vi "setRowsColor.vi"(8 "error in (no error)":errorcluster, 10 "rowsColor":u32[](array[numeric]), 11 "reference in":refnum<class "excelFile.lvclass">) -> (0 "error out":errorcluster, 3 "reference out":refnum<class "excelFile.lvclass">)   [LabVIEW 2016, in "excelFile.lvclass"]
uses:
  excelFile.lvclass
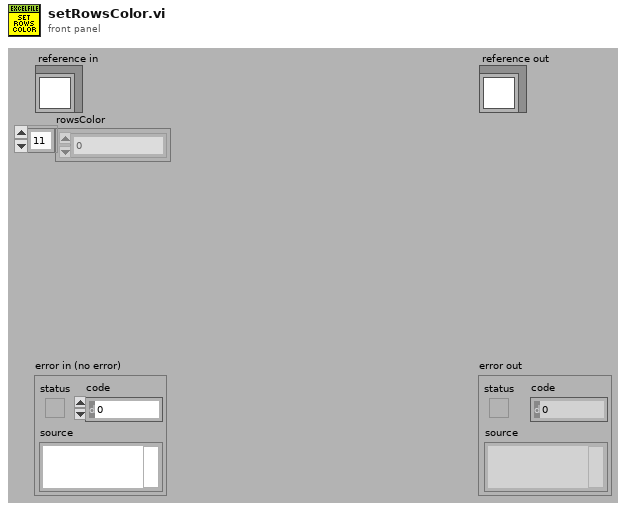
[diagram p1: front panel]
types:
  T1 = typedef "excelFile.lvclass/ObjectAttributesRef.ctl" = refnum<data-value>
  T2 = typedef "excelFile.lvclass/ObjectAttributes.ctl" = cluster{"MyAttribute":dbl, "path":string, "Refnum Excel":cluster{"Excel._Application":refnum<k7>, "Workbooks":refnum<k7>, "Open":refnum<k7>}, "data":string[][][], "save":bool, "fileType":T3, "rowsColor":u32[], "python_ref":refnum<class "python.lvclass">, "items_rows":i32[], "excel_range":i32[][], "TSR":cluster{"number":string, "TSR_path":path, "service_path":path, "email_to":string}, "excel_already_opened?":bool, "file_already_opened?":bool, "excel_protected_opened?":bool, "Refnum Cluster Worksheets":cluster{"Excel._Application":refnum<k7>, "Workbooks":refnum<k7>, "Open":refnum<k7>, "Worksheets":refnum<k7>, "Excel._Worksheet":refnum<k7>}, "#_rows_defective":i32, "#_rows_spare":i32}
  T3 = typedef "excelFile.lvclass/fileType.ctl" = enum16{"devices", "items", "partsTracking", "TSR"}
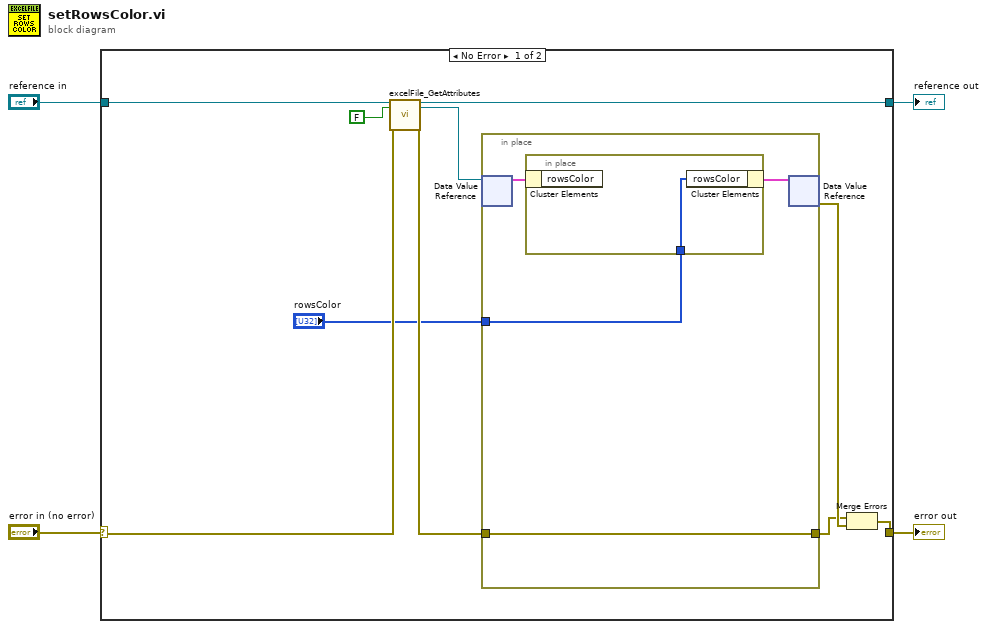
[diagram p0: block diagram]
diagram:
  n1 = case shown="No Error" "error in (no error)" {
    selector: "error in (no error)" -> [w9 w21]
    tunnel: [w14 w21] -> w3
    tunnel: [w7 w20] -> w1
    tunnel: "reference in" -> [w11 w20]
    frame No Error {
      n2 = call "excelFile_GetAttributes.vi"("reference in"=w11, "return data? (T)"=FALSE, "error in (no error)"=w9) -> ("reference out"=w7:refnum<class "excelFile.lvclass">, "attributes ref"=w6:T1, "error out"=w8:errorcluster)  [unwired: 13 in, 1 out]
      n3 = in-place {
        in-place-border: w8 -> [w16]
        in-place-border: [w16] -> w12
        in-place-border: "rowsColor" -> [w15]
        n4 = in-place-dvr #1(w6) -> (w17:T2)  [unwired: 1 out]
        n5 = in-place {
          in-place-border: w15 -> [w19]
          n6 = in-place-cluster #2(w17) -> ()  [unwired: 1 out]
          n7 = in-place-cluster #2("rowsColor"=w19) -> (w18:T2)
        }
        n8 = in-place-dvr #1(w18) -> (w13:errorcluster)  [unwired: 1 out]
      }
      n9 = Merge Errors(w12, w13) -> (w14:errorcluster)
    }
    frame Error {
    }
  }
  "error out" <- w3
  "reference out" <- w1
